vi "Unicode Conversion Example.vi"() -> ()   [LabVIEW 2020]
uses:
  Unicode/Controls/String Encoding.ctl
  Types/UTF-8 String/UTF-8 String.lvclass/UTF-8 String.ctl
  Dialog & User Interface/Polymorphic VIs/Write Control Text/Write String Value (UTF-8 String).vi
  Private/Conversion/Text to UTF-8.vi
  Private/Conversion/Polymorphic VIs/Text to UTF-8 (LabVIEW String).vi
  Dialog & User Interface/Polymorphic VIs/Write Control Text/Write String Value (UTF-8 String).vi/5206cb6b-04fb-41f5-a37e-29c14f142303.vi
  Private/Conversion/Text as Encoded String.vi
  Private/Conversion/Polymorphic VIs/Text as Encoded String (UTF-8 String).vi
  Types/UTF-8 String/Read Encoded UTF-8 String.vi
  Unicode/Detect String Encoding.vi
  Private/Conversion/Encoded UTF-16LE String to Encoded UTF-8 String.vi
  Private/Conversion/Encoded UTF-8 String to Encoded UTF-16LE String.vi
  Private/User Interface/Write String.vi
  Types/UTF-8 String/UTF-8 String.lvclass
  G-Unicode.lvlib
panel:
  out "ANSI -> UTF-16LE (Encoded)":string
  out "UTF-8 -> UTF-16LE (Encoded)":string
  out "UTF-8  -> UTF-16LE":string
  out "ANSI -> UTF-16LE":string
  out "UTF-16LE":string
  out "UTF-8":string
  out "ANSI":string
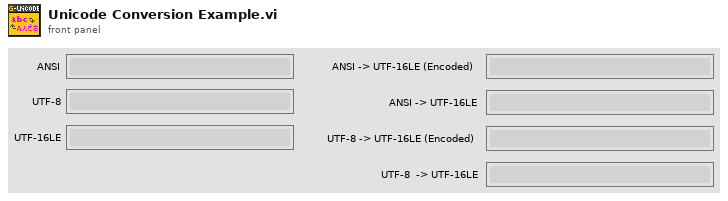
[diagram p1: front panel]
types:
  T1 = typedef "G-Unicode.lvlib/String Encoding.ctl" = enum16{"ANSI", "UTF-8", "UTF-16LE", "UTF-16BE", "Unknown"}
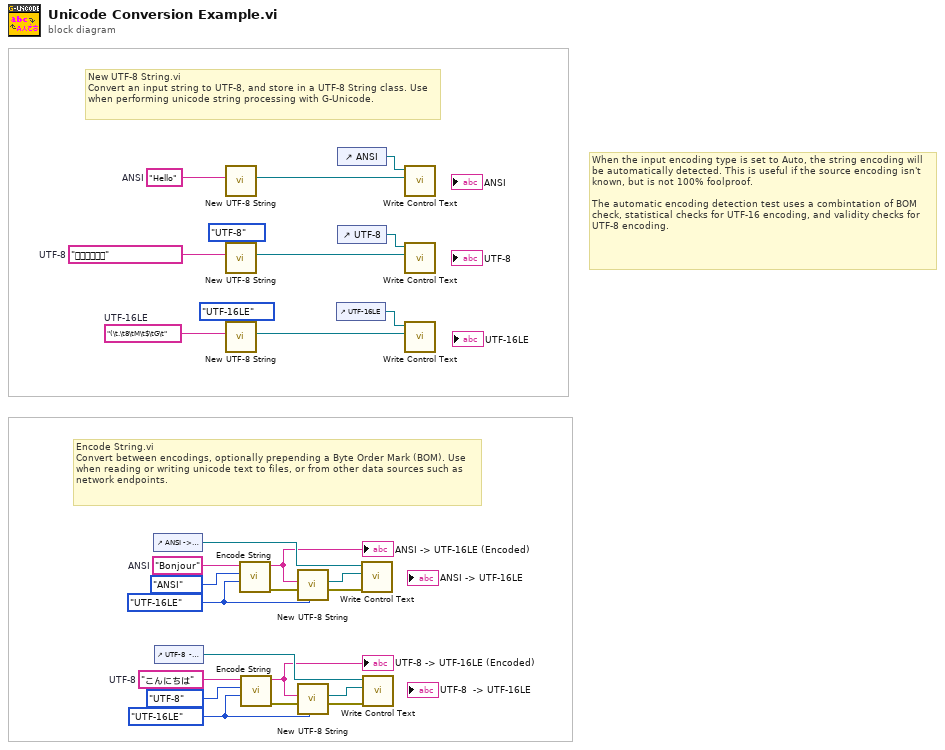
[diagram p0: block diagram]
diagram:
  w6 = String_Encoding."UTF-16LE" ("Output Encoding (UTF-16LE)")
  w12 = "Bonjour"  # ANSI
  w3 = String_Encoding."UTF-16LE" ("Output Encoding (UTF-16LE)")
  w16 = "こんにちは"  # UTF-8
  w24 = "(\t.\t8\tM\t$\tG\t"  # UTF-16LE
  w25 = "नमस्ते"  # UTF-8
  w27 = "Hello"  # ANSI
  # "When the input encoding type is set to Auto, the string encoding will be automatically detected. This is useful if the source encoding isn't known, but is not 100% foolproof.\n\nThe automatic encoding detection test uses a combintation of BOM check, statistical checks for UTF-16 encoding, and validity checks for UTF-8 encoding."
  # "Encode String.vi\nConvert between encodings, optionally prepending a Byte Order Mark (BOM). Use when reading or writing unicode text to files, or from other data sources such as network endpoints."
  # "New UTF-8 String.vi\nConvert an input string to UTF-8, and store in a UTF-8 String class. Use when performing unicode string processing with G-Unicode."
  n1 = control-ref of="ANSI -> UTF-16LE"() -> (w11:refnum<vi>)
  n2 = control-ref of="UTF-8  -> UTF-16LE"() -> (w14:refnum<vi>)
  n3 = call "New UTF-8 String.vi"("String"=w27) -> ("UTF-8 String"=w22:refnum<class "UTF-8 String.lvclass">)  [unwired: 9 in, 1 out]
  n4 = call "New UTF-8 String.vi"("Input Encoding (ANSI)"=String_Encoding."UTF-8", "String"=w25) -> ("UTF-8 String"=w19:refnum<class "UTF-8 String.lvclass">)  [unwired: 8 in, 1 out]
  n5 = call "New UTF-8 String.vi"("Input Encoding (ANSI)"=String_Encoding."UTF-16LE", "String"=w24) -> ("UTF-8 String"=w18:refnum<class "UTF-8 String.lvclass">)  [unwired: 8 in, 1 out]
  n6 = call "Encode String.vi"("Output Encoding (UTF-16LE)"=w6, "Input Encoding (ANSI)"=String_Encoding."ANSI", "String in"=w12) -> ("error out"=w8:errorcluster, "String out"=w10:string)  [unwired: 7 in]
  "ANSI -> UTF-16LE (Encoded)" <- w10
  n7 = call "Encode String.vi"("Output Encoding (UTF-16LE)"=w3, "Input Encoding (ANSI)"=String_Encoding."UTF-8", "String in"=w16) -> ("error out"=w5:errorcluster, "String out"=w2:string)  [unwired: 7 in]
  "UTF-8 -> UTF-16LE (Encoded)" <- w2
  n8 = call "New UTF-8 String.vi"("Input Encoding (ANSI)"=w6, "error in"=w8, "String"=w10) -> ("error out"=w7:errorcluster, "UTF-8 String"=w9:refnum<class "UTF-8 String.lvclass">)  [unwired: 7 in]
  n9 = call "New UTF-8 String.vi"("Input Encoding (ANSI)"=w3, "error in"=w5, "String"=w2) -> ("error out"=w4:errorcluster, "UTF-8 String"=w1:refnum<class "UTF-8 String.lvclass">)  [unwired: 7 in]
  n10 = control-ref of="UTF-16LE"() -> (w17:refnum<vi>)
  n11 = control-ref of="ANSI"() -> (w21:refnum<vi>)
  n12 = control-ref of="UTF-8"() -> (w20:refnum<vi>)
  n13 = call-poly "Write Control Text.vi"("error in"=w7, "Value"=w9, "Control Ref"=w11) -> ()  [unwired: 8 in, 1 out]
  n14 = call-poly "Write Control Text.vi"("error in"=w4, "Value"=w1, "Control Ref"=w14) -> ()  [unwired: 8 in, 1 out]
  n15 = call-poly "Write Control Text.vi"("Value"=w22, "Control Ref"=w21) -> ()  [unwired: 9 in, 1 out]
  n16 = call-poly "Write Control Text.vi"("Value"=w19, "Control Ref"=w20) -> ()  [unwired: 9 in, 1 out]
  n17 = call-poly "Write Control Text.vi"("Value"=w18, "Control Ref"=w17) -> ()  [unwired: 9 in, 1 out]
